vi "Start.vi"(8 "error in (no error)":errorcluster, 11 "Actor API in":refnum<class "Actor API.lvclass">) -> (0 "error out":errorcluster, 3 "Actor API out":refnum<class "Actor API.lvclass">)   [LabVIEW 2022 SP3, in "Artifex.lvlib" / "Actor API.lvclass"]
uses:
  Actor API.lvclass
  Actor API.lvclass/Actor API.ctl
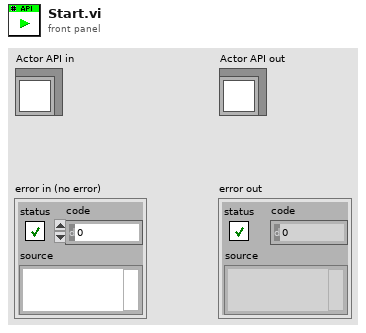
[diagram p1: front panel]
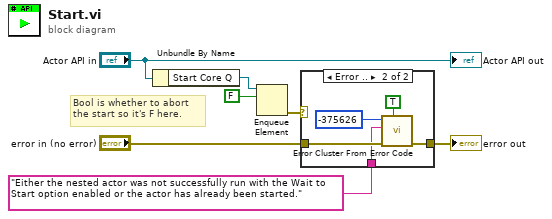
[diagram p0: block diagram]
diagram:
  # "Bool is whether to abort the start so it's F here."
  n1 = Unbundle By Name("Actor API in") -> ("Start Core Q"=w6:refnum<queue>)
  n2 = Enqueue Element(queue=w6, element=FALSE) -> (error out=w4:errorcluster)  [unwired: 2 in, 2 out]
  n3 = case shown="Error .." w4 {
    tunnel: "error in (no error)" -> [w8 w13]
    tunnel: [w8 w12] -> w2
    tunnel: "Either the nested actor was not successfully run with the Wait to Start option enabled or the actor has already been started." -> [_ w9]
    frame No Error {
    }
    frame Error {
      n4 = call <vilib>:"Error Cluster From Error Code.vi"("show call chain? (False)"=TRUE, "error in (no error)"=w13, "error message (\"\")"=w9, "error code (0)"=-375626) -> ("error out"=w12:errorcluster)  [unwired: 5 in]
    }
  }
  "error out" <- w2
  "Actor API out" <- "Actor API in"
